vi "S&E Error String.vi"(2 "Elevated priority":bool, 7 "Content":variant, 9 "error in":errorcluster) -> (8 "format string":string, 10 "error out":errorcluster)   [LabVIEW 2011]
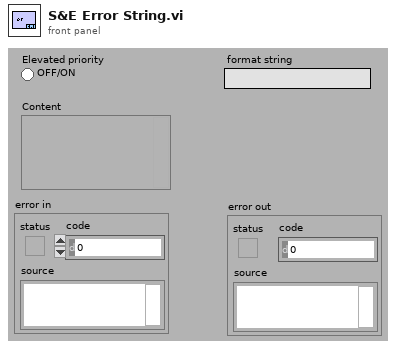
[diagram p1: front panel]
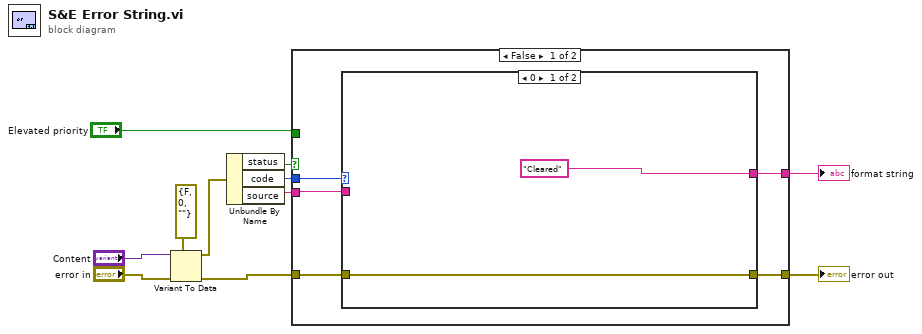
[diagram p0: block diagram]
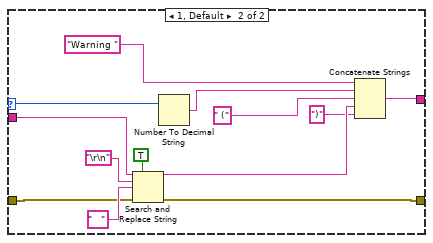
[diagram p2: hidden frame]
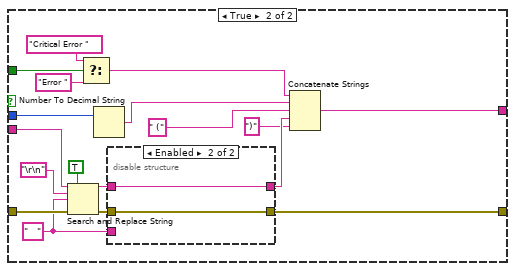
[diagram p3: hidden frame]
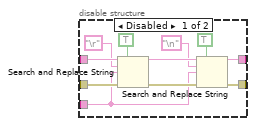
[diagram p4: hidden frame]
diagram:
  n1 = Variant To Data(error in="error in", type=errorcluster {"status"=FALSE, "code"=0, "source"=""} ("error in (no error)"), Variant="Content") -> (data=w1:errorcluster, error out=w2:errorcluster)
  n2 = Unbundle By Name(w1) -> ("status"=w3:bool, "code"=w4:i32, "source"=w5:string)
  n3 = case shown="False" w3 {
    tunnel: w4 -> [w13 w49]
    tunnel: w5 -> [w12 w45]
    tunnel: [w16 w48] -> w11
    tunnel: w2 -> [w14 w38]
    tunnel: [w15 w37] -> w9
    tunnel: "Elevated priority" -> [_ w36]
    frame False {
      n4 = case shown="0" w13 {
        selector: w13 -> [_ w21]
        tunnel: ["Cleared" ("format string") w19] -> w16
        tunnel: [w17 w22] -> w15
        tunnel: w14 -> [w17 w23]
        tunnel: w12 -> [_ w20]
        frame 0 {
        }
        frame 1, Default {
          n5 = Search and Replace String(replace all?=TRUE ("replace all? (F)"), input string=w20, search string="\r\n", replace string="   " ("format string"), error in=w23) -> (result string=w27:string, error out=w22:errorcluster)  [unwired: 3 in, 2 out]
          n6 = Number To Decimal String(number=w21) -> (decimal integer string=w31:string)  [unwired: 1 in]
          n7 = Concatenate Strings("Warning " ("format string"), w31, " (" ("string"), w27, ")" ("string")) -> (w19:string)
        }
      }
    }
    frame True {
      w32 = "   " ("format string")
      n8 = Search and Replace String(replace all?=TRUE ("replace all? (F)"), input string=w45, search string="\r\n", replace string=w32, error in=w38) -> (result string=w43:string, error out=w42:errorcluster)  [unwired: 3 in, 2 out]
      n9 = Select(t="Critical Error ", s=w36, f="Error " ("format string")) -> (s? t:f=w34:string)
      n10 = Number To Decimal String(number=w49) -> (decimal integer string=w47:string)  [unwired: 1 in]
      n11 = disable-structure shown="Enabled" {
        disable-tunnel: w43 -> [w58 w62]
        disable-tunnel: [w54 w62] -> w40
        disable-tunnel: w42 -> [w53 w61]
        disable-tunnel: [w51 w61] -> w37
        disable-tunnel: w32 -> [w50 _]
        frame Disabled {
          n12 = Search and Replace String(replace all?=TRUE ("replace all? (F)"), input string=w58, search string="\r", replace string=w50, error in=w53) -> (result string=w57:string, error out=w52:errorcluster)  [unwired: 3 in, 2 out]
          n13 = Search and Replace String(replace all?=TRUE ("replace all? (F)"), input string=w57, search string="\n", replace string=w50, error in=w52) -> (result string=w54:string, error out=w51:errorcluster)  [unwired: 3 in, 2 out]
        }
        frame Enabled {
        }
      }
      n14 = Concatenate Strings(w34, w47, " (" ("string"), w40, ")" ("string")) -> (w48:string)
    }
  }
  "format string" <- w11
  "error out" <- w9
